vi "Set Diverter Port.vi"(6 "wait for reply (T)":bool=TRUE, 8 "error in (no error)":errorcluster, 9 "Diverter Port":T2, 10 "Diverter Location":T3) -> (0 "error out":errorcluster, 1 "timed out?":bool, 2 "Reply Payload":T1)   [LabVIEW 2020, in "Spectrometer.lvlib"]
doc: "_____\nCreated using Delacor QMH Event Scripter 5.0.0.112."
uses:
  Spectrometer.lvlib
  SpectraPro-LabVIEW-Driver/Libraries/Types/Diverter Location.ctl
  SpectraPro-LabVIEW-Driver/Libraries/Types/Diverter Port.ctl
  Set Diverter Port (Reply Payload)--cluster.ctl
  Set Diverter Port Argument--cluster.ctl
  SpectraPro-LabVIEW-Driver/SpectraPro.lvlib
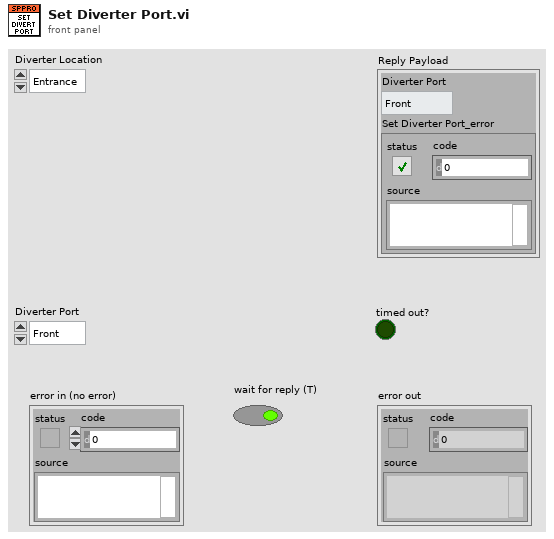
[diagram p1: front panel]
types:
  T1 = typedef "Spectrometer.lvlib/Set Diverter Port (Reply Payload)--cluster.ctl" = cluster{"Diverter Port":T2, "Set Diverter Port_error":errorcluster}
  T2 = typedef "SpectraPro.lvlib/Diverter Port.ctl" = enum16{"Front", "Side"}
  T3 = typedef "Diverter Location.ctl" = enum16{"Entrance", "Exit"}
  T4 = typedef "Spectrometer.lvlib/Set Diverter Port Argument--cluster.ctl" = cluster{"Diverter Location":T3, "Diverter Port":T2, "Wait Notifier":refnum<notifier>, "wait for reply":bool}
  T5 = typedef "Spectrometer.lvlib/Request Events--cluster.ctl" = cluster{"Stop Module":refnum<user-event>, "Show Panel":refnum<user-event>, "Hide Panel":refnum<user-event>, "Get Module Execution Status":refnum<user-event>, "Show Diagram":refnum<user-event>, "Set Wavelength":refnum<user-event>, "Set Slit Width":refnum<user-event>, "Set Grating":refnum<user-event>, "Get Module Data":refnum<user-event>, "Set Diverter Port":refnum<user-event>}
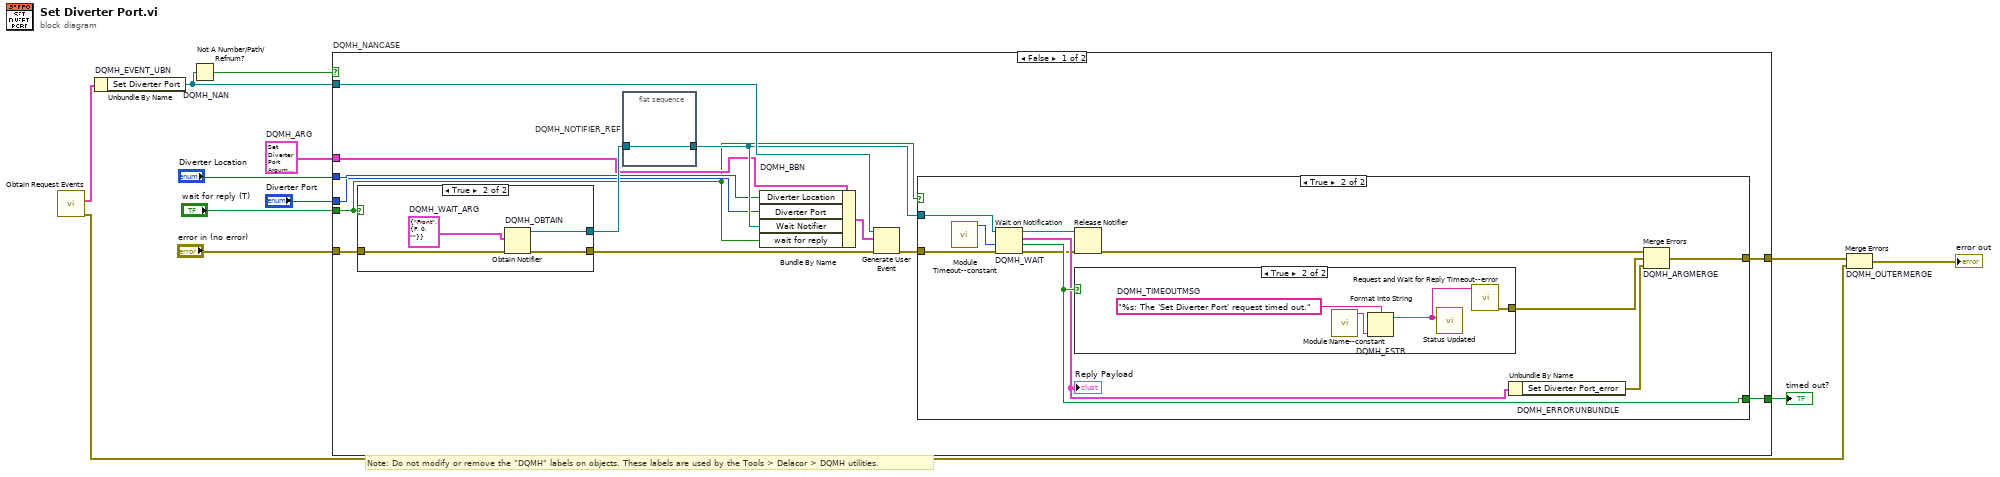
[diagram p0: block diagram]
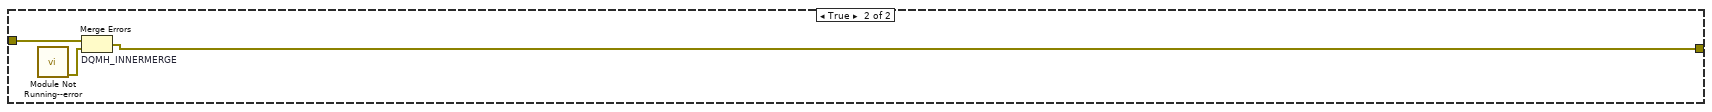
[diagram p5: hidden frame]
diagram:
  w6 = T4 {"Diverter Location"=enum."Entrance", "Diverter Port"=enum."Front", "Wait Notifier"=refnum, "wait for reply"=FALSE}  # DQMH_ARG
  # "Note: Do not modify or remove the \"DQMH\" labels on objects. These labels are used by the Tools > Delacor > DQMH utilities."
  n1 = call "Obtain Request Events.vi"() -> ("error out"=w2:errorcluster, "Spectrometer Request Events"=w1:T5)  [unwired: 10 in]
  n2 = Unbundle By Name "DQMH_EVENT_UBN"(w1) -> ("Set Diverter Port"=w10:refnum<user-event>)
  n3 = Not A Number/Path/Refnum? "DQMH_NAN"(number/path/refnum=w10) -> (NaN/Path/Refnum?=w9:bool)
  n4 = case "DQMH_NANCASE" shown="False" w9 {
    tunnel: "error in (no error)" -> [w25 w50]
    tunnel: w10 -> [w23 _]
    tunnel: [w20 w49] -> w7
    tunnel: [w21 _] -> w8
    tunnel: w6 -> [w16 _]
    tunnel: "Diverter Location" -> [w15 _]
    tunnel: "Diverter Port" -> [w14 _]
    tunnel: "wait for reply (T)" -> [w13 _]
    frame False {
      n5 = case shown="True" w13 {
        tunnel: w25 -> [w43 w47]
        tunnel: [w43 w46] -> w22
        tunnel: [_ w44] -> w18
        frame False {
        }
        frame True {
          w45 = T1 {"Diverter Port"=enum."Front", "Set Diverter Port_error"={"status"=FALSE, "code"=0, "source"=""}}  # DQMH_WAIT_ARG
          n6 = Obtain Notifier "DQMH_OBTAIN"(notification data type=w45, error in (no error)=w47) -> (notifier out=w44:refnum<notifier>, error out=w46:errorcluster)  [unwired: 2 in, 1 out]
        }
      }
      n7 = flat-sequence "DQMH_NOTIFIER_REF" {
        tunnel: w18 -> [w26]
        tunnel: [w26] -> w17
        frame #0 {
        }
      }
      n8 = Bundle By Name "DQMH_BBN"(cluster=w16, "Diverter Location"=w15, "Diverter Port"=w14, "Wait Notifier"=w17, "wait for reply"=w13) -> (w19:T4)
      n9 = Generate User Event(user event=w23, event data cluster=w19, error in=w22) -> (error out=w24:errorcluster)  [unwired: 1 in, 1 out]
      n10 = case shown="True" w13 {
        tunnel: w24 -> [w27 w38]
        tunnel: w17 -> [_ w37]
        tunnel: [_ w35] -> w21
        tunnel: [w27 w34] -> w20
        frame False {
        }
        frame True {
          n11 = call "Module Timeout--constant.vi"() -> ("Module Timeout"=w28:i32)  [unwired: 11 in]
          n12 = Wait on Notification "DQMH_WAIT"(notifier=w37, timeout in ms (-1)=w28, error in (no error)=w38) -> (notifier out=w36:refnum<notifier>, notification=w33:T1, timed out?=w35:bool, error out=w32:errorcluster)  [unwired: 1 in]
          "Reply Payload" <- w33
          n13 = Release Notifier(notifier=w36, error in (no error)=w32) -> (error out=w31:errorcluster)  [unwired: 1 in, 2 out]
          n14 = case shown="True" w35 {
            tunnel: [_ w40] -> w29
            frame False {
            }
            frame True {
              w42 = "%s: The 'Set Diverter Port' request timed out."  # DQMH_TIMEOUTMSG
              n15 = call "Module Name--constant.vi"() -> ("Module Name"=w39:string)  [unwired: 11 in]
              n16 = Format Into String "DQMH_FSTR"(format string=w42, w39) -> (resulting string=w41:string)  [unwired: 2 in, 1 out]
              n17 = call "Status Updated.vi"("Status"=w41) -> ()  [unwired: 10 in, 1 out]
              n18 = call "Request and Wait for Reply Timeout--error.vi"("Error Message"=w41) -> ("error out"=w40:errorcluster)  [unwired: 10 in]
            }
          }
          n19 = Unbundle By Name "DQMH_ERRORUNBUNDLE"(w33) -> ("Set Diverter Port_error"=w30:errorcluster)
          n20 = Merge Errors "DQMH_ARGMERGE"(w31, w29, w30) -> (w34:errorcluster)
        }
      }
    }
    frame True {
      n21 = call "Module Not Running--error.vi"() -> ("error out"=w48:errorcluster)  [unwired: 11 in]
      n22 = Merge Errors "DQMH_INNERMERGE"(w50, w48) -> (w49:errorcluster)
    }
  }
  "timed out?" <- w8
  n23 = Merge Errors "DQMH_OUTERMERGE"(w7, w2) -> (→"error out":errorcluster)
